vi "Loop_ACT_Drive.vi"() -> ()   [LabVIEW 2017]
uses:
  TypeDef/CLUSTER_Drive_HW_SRX_Status.ctl
  TypeDef/CLUSTER_4296_SRX_Status.ctl
  TypeDef/CLUSTER_SRX_Status Data.ctl
  TypeDef/CLUSTER_SRX_Encoder Data.ctl
  TypeDef/CLUSTER_SRX_PWM Data.ctl
  TypeDef/CLUSTER_SRX_Analog Data.ctl
  TypeDef/CLUSTER_SRX_Limit Switch Data.ctl
  TypeDef/CLUSTER_SRX_Profile Data.ctl
  TypeDef/ENUM_Drive_ACT Loop_Mode.ctl
  TypeDef/CLUSTER_Left and Right.ctl
  System Drivers/Phoenix-LabVIEW/Motor Controller/Controls/CTRE_Phoenix_MotorControl_FeedbackDevice.ctl
  System Drivers/Phoenix-LabVIEW/Motor Controller/Controls/CTRE_Phoenix_MotorControl_NeutralMode.ctl
  <vilib>/Rock Robotics/WPI/RobotDrive/WPI_RobotDriveOpen4MotorWithExistingMotors.vi
  _SHARE ALL/Global Share All/Global_STOP.vi
  Global_SM Write_Data Out.vi
  Global_ACT Write_Data Out.vi
  Drive Code/RoboRio Code/Systems/WCDrive2018/WCDrive2018.lvlib
  Drive Code/RoboRio Code/Systems/WCDrive2018/Cluster_WCDrive_SetupData.ctl
panel:
  in  "Zero Encoder":bool
  in  "D":dbl
  in  "I":dbl
  in  "P":dbl
  out "Right Data":dbl
  out "Left Data":dbl
  out "Cycle Time (S)":dbl format="%.3g"
  in  "Target Time(ms)":u32=50
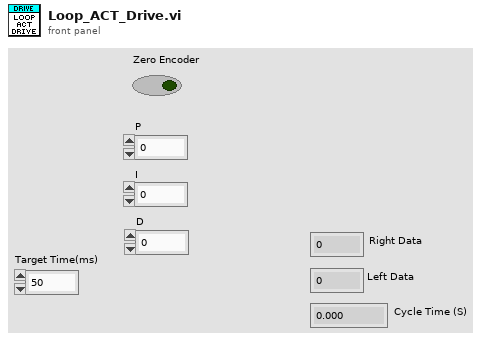
[diagram p1: front panel]
types:
  T1 = typedef "CTRE_Phoenix_MotorControl_NeutralMode.ctl" = enum8{"EEPROMSetting", "Override to Coast", "Override to Brake"}
  T2 = typedef "CTRE_Phoenix_MotorControl_FeedbackDevice.ctl" = i8
  T3 = typedef "CLUSTER_Left and Right.ctl" = cluster{"Left":dbl, "Right":dbl}
  T4 = typedef "ENUM_Drive_ACT Loop_Mode.ctl" = enum16{"Stop", "Position", "VBus", "Profile"}
  T5 = typedef "CLUSTER_Drive_HW_SRX_Status.ctl" = cluster{"Rear Left":T6, "Rear Right":T6, "Front Left":T6, "Front Right":T6}
  T6 = typedef "CLUSTER_4296_SRX_Status.ctl" = cluster{"Status":T7, "Encoder":T8, "PWM ":T9, "Analog":T10, "Limit Switches":T11, "Profile":T12}
  T7 = typedef "CLUSTER_SRX_Status Data.ctl" = cluster{"Module Enabled":bool, "Current Profile Slot Select":dbl, "Brake is Enabled":bool, "Applied Throttle":dbl, "Current":dbl, "Battery Voltage":dbl, "Sticky Fault - Under Voltage":bool, "Temperature (C)":dbl, "Sticky Fault - Over Temp":bool, "CAN Error":errorcluster, "Control 5 Is Supported":bool}
  T8 = typedef "CLUSTER_SRX_Encoder Data.ctl" = cluster{"Closed Loop Error":dbl, "Sensor Position":dbl, "Sensor Velocity":dbl, "Encoder Position":dbl, "Encoder Velocity":dbl, "Encoder Index Count":dbl, "Encoder A Pin State":bool, "Encoder B Pin State":bool, "Encoder Index Pin State":bool, "Pos Div 8":bool, "Vel Div 4":bool}
  T9 = typedef "CLUSTER_SRX_PWM Data.ctl" = cluster{"Closed Loop Error":dbl, "Pulse Width Position":i32, "Pulse Width Velocity":i32, "Pulse Width Rise To Rise (us)":i32, "Pulse Width Rise To Fall (us)":i32}
  T10 = typedef "CLUSTER_SRX_Analog Data.ctl" = cluster{"Closed Loop Error":dbl, "Analog In":dbl, "Analog In Velocity":dbl}
  T11 = typedef "CLUSTER_SRX_Limit Switch Data.ctl" = cluster{"Forward Limit Switch Closed":bool, "Reverse Limit Switch Closed":bool, "Sticky Fault - Forward Limit":bool, "Sticky Fault - Reverse Limit":bool, "Sticky Fault - Forward Soft Limit":bool, "Sticky Fault - Reverse Soft Limit":bool}
  T12 = typedef "CLUSTER_SRX_Profile Data.ctl" = cluster{"Mot Prof Active Is Under Run":bool, "Mot Prof Active Has Under Run":bool, "Mot Prof Active Is Last":bool, "Mot Prof Active Velocity Only":bool, "Mot Prof Active Is Valid":bool, "Mot Prof Buffer Is Full":bool, "Mot Prof Active Profile Slot Select":i32, "Mot Prof NextID":i32, "Mot Prof Count":i32, "Mot Prof Active Velocity":dbl, "Mot Prof Active Position":dbl, "Mot Prof Output Enable":i32}
  T13 = typedef "Cluster_WCDrive_SetupData.ctl" = cluster{"Left Master":u8, "Invert Left Master":bool, "Left Slave":u8, "Invert Left Slave":bool, "Right Master":u8, "Invert Right Master":bool, "Right Slave":u8, "Invert Right Slave":bool, "Invert Left Encoder":bool, "Invert Right Encoder":bool}
  T14 = typedef "WPI_MotorControlDeviceRef.ctl" = cluster{"DeviceStatus":errorcluster, "Type":T15, "PWM":cluster{"PWM Channel":T16, "DeadBand":T17}, "CAN":cluster{"Device Number":u8, "SetOutput VI Ref":variant, "GetOutput VI Ref":variant, "Enable VI Ref":variant, "Disable VI Ref":variant, "Data":variant}, "Invert":bool, "DIO PWM":cluster{"PWM \"Enable\" Channel":T16, "DIOChannel":T18, "PWM Rate":dbl}}
  T15 = typedef "WPI_MotorControlType.ctl" = enum16{"PWM", "CAN", "DIO PWM"}
  T16 = typedef "FPGA_DIOPWMChannel.ctl" = enum8{"PWM 0", "PWM 1", "PWM 2", "PWM 3", "PWM 4", "PWM 5", "PWM 6", "PWM 7", "PWM 8", "PWM 9", "PWM MXP 0", "PWM MXP 1", "PWM MXP 2", "PWM MXP 3", "PWM MXP 4", "PWM MXP 5", "PWM MXP 6", "PWM MXP 7", "PWM MXP 8", "PWM MXP 9", "Invalid"}
  T17 = typedef "WPI_PWMDeadband.ctl" = cluster{"Name":string, "maxPositivePwm":i32, "minPositivePwm":i32, "centerPwm":i32, "maxNegativePwm":i32, "minNegativePwm":i32, "angularRange":u16}
  T18 = typedef "FPGA_DIOChannel.ctl" = enum8{"DIO 0", "DIO 1", "DIO 2", "DIO 3", "DIO 4", "DIO 5", "DIO 6", "DIO 7", "DIO 8", "DIO 9", "DIO MXP 0", "DIO MXP 1", "DIO MXP 2", "DIO MXP 3", "DIO MXP 4", "DIO MXP 5", "DIO MXP 6", "DIO MXP 7", "DIO MXP 8", "DIO MXP 9", "DIO MXP 10", "DIO MXP 11", "DIO MXP 12", "DIO MXP 13", "DIO MXP 14", "DIO MXP 15", "SPI Port CS1", "SPI Port CS2", "SPI Port CS3", "SPI Port MISO", "SPI Port MOSI", "Invalid"}
  T19 = typedef "WPI_RobotDriveDevRef.ctl" = cluster{"DevStatus":errorcluster, "Motors[]":T14[], "Square Inputs":bool, "Max Output":dbl}
  T20 = cluster{"RobotDriveDevRef":T19, "Target Time(ms)":u32, "Current Time":timestamp, "Previous Time":timestamp, "Cycle Time (S)":dbl, "SRX_Status":T5, "Mode":T4, "VBus":T3, "Cruise RPM":dbl, "MAX Velocity\n":dbl, "Encoder Target Position":i32, "Zero Encoder":bool}
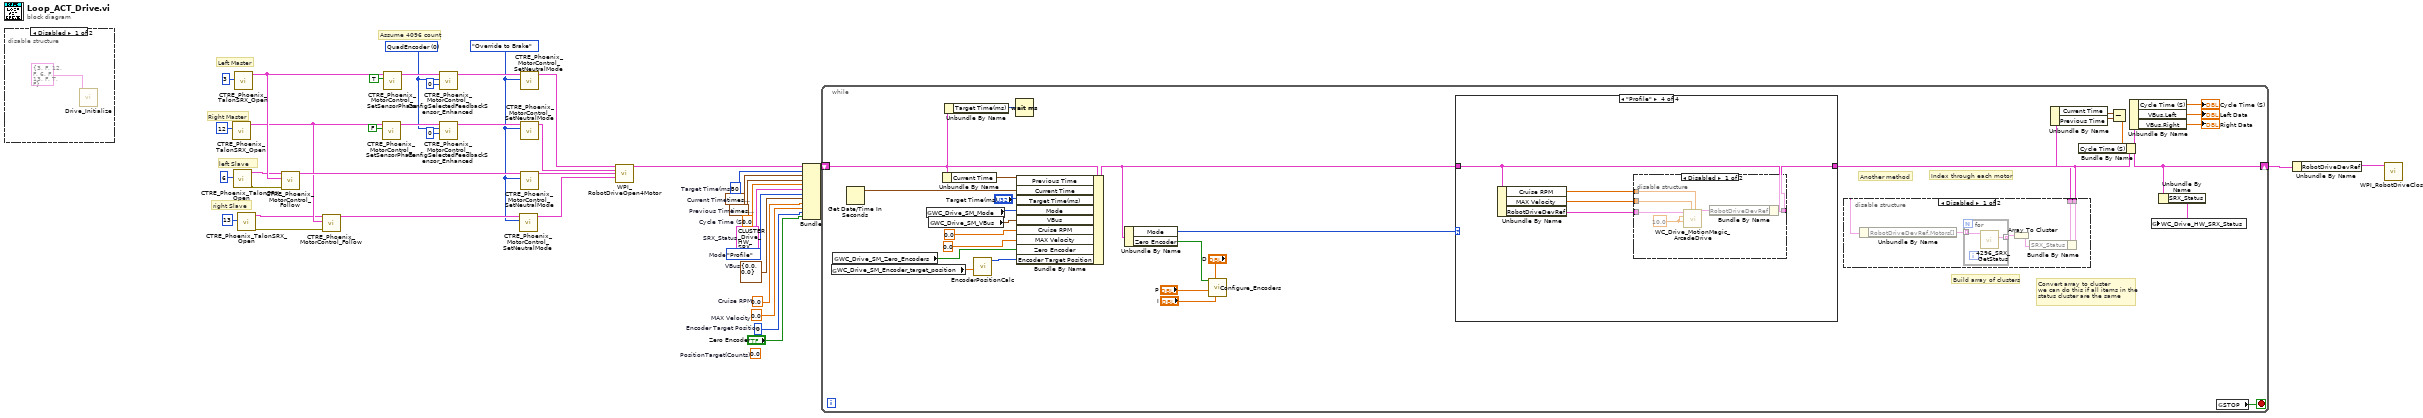
[diagram p0: block diagram]
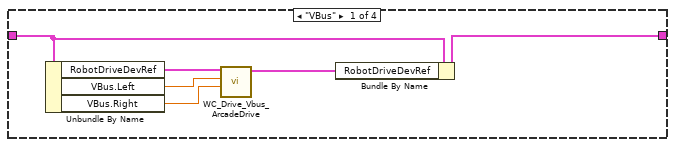
[diagram p4: hidden frame]
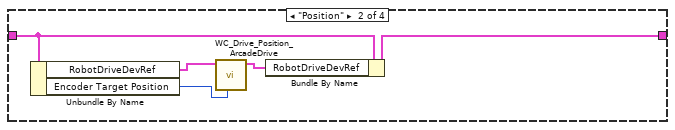
[diagram p5: hidden frame]
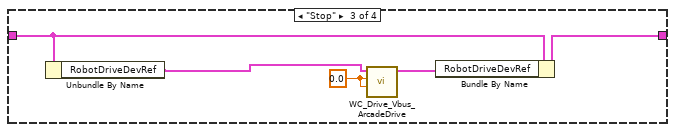
[diagram p6: hidden frame]
diagram:
  w14 = CTRE_Phoenix_MotorControl_NeutralMode."Override to Brake" ("Motor Control Neutral Mode")
  w17 = T2 0 items=["None"=-1, "QuadEncoder"=0, "Analog"=2, "Tachometer"=4, "Pulse Width Encoded Position"=8, "Sensor Sum (S0 + S1)"=9, "Sensor Difference (D0 - D1)"=10, "Remote Source 0"=11, "Remote Source 1"=12, "Software Emulated"=15] ("Feedback Device")
  (unwired) 0.0  # PositionTarget(Counts)
  w29 = 0  # Encoder Target Position
  w30 = 0.0  # MAX Velocity
  w31 = 0.0  # Cruise RPM
  w32 = T3 {"Left"=0.0, "Right"=0.0}  # VBus
  w33 = ENUM_Drive_ACT_Loop_Mode."Profile"  # Mode
  w34 = T5 {"Rear Left"={"Status"={"Module Enabled"=FALSE, "Current Profile Slot Select"=0.0, "Brake is Enabled"=FALSE, "Applied Throttle"=0.0, "Current"=0.0, "Battery Voltage"=0.0, "Sticky Fault - Under Voltage"=FALSE, "Temperature (C)"=0.0, "Sticky Fault - Over Temp"=FALSE, "CAN Error"={"status"=FALSE, "code"=0, "source"=""}, "Control 5 Is Supported"=FALSE}, "Encoder"={"Closed Loop Error"=0.0, "Sensor Position"=0.0, "Sensor Velocity"=0.0, "Encoder Position"=0.0, "Encoder Velocity"=0.0, "Encoder Index Count"=0.0, "Encoder A Pin State"=FALSE, "Encoder B Pin State"=FALSE, "Encoder Index Pin State"=FALSE, "Pos Div 8"=FALSE, "Vel Div 4"=FALSE}, "PWM "={"Closed Loop Error"=0.0, "Pulse Width Position"=0, "Pulse Width Velocity"=0, "Pulse Width Rise To Rise (us)"=0, "Pulse Width Rise To Fall (us)"=0}, "Analog"={"Closed Loop Error"=0.0, "Analog In"=0.0, "Analog In Velocity"=0.0}, "Limit Switches"={"Forward Limit Switch Closed"=FALSE, "Reverse Limit Switch Closed"=FALSE, "Sticky Fault - Forward Limit"=FALSE, "Sticky Fault - Reverse Limit"=FALSE, "Sticky Fault - Forward Soft Limit"=FALSE, "Sticky Fault - Reverse Soft Limit"=FALSE}, "Profile"={"Mot Prof Active Is Under Run"=FALSE, "Mot Prof Active Has Under Run"=FALSE, "Mot Prof Active Is Last"=FALSE, "Mot Prof Active Velocity Only"=FALSE, "Mot Prof Active Is Valid"=FALSE, "Mot Prof Buffer Is Full"=FALSE, "Mot Prof Active Profile Slot Select"=0, "Mot Prof NextID"=0, "Mot Prof Count"=0, "Mot Prof Active Velocity"=0.0, "Mot Prof Active Position"=0.0, "Mot Prof Output Enable"=0}}, "Rear Right"={"Status"={"Module Enabled"=FALSE, "Current Profile Slot Select"=0.0, "Brake is Enabled"=FALSE, "Applied Throttle"=0.0, "Current"=0.0, "Battery Voltage"=0.0, "Sticky Fault - Under Voltage"=FALSE, "Temperature (C)"=0.0, "Sticky Fault - Over Temp"=FALSE, "CAN Error"={"status"=FALSE, "code"=0, "source"=""}, "Control 5 Is Supported"=FALSE}, "Encoder"={"Closed Loop Error"=0.0, "Sensor Position"=0.0, "Sensor Velocity"=0.0, "Encoder Position"=0.0, "Encoder Velocity"=0.0, "Encoder Index Count"=0.0, "Encoder A Pin State"=FALSE, "Encoder B Pin State"=FALSE, "Encoder Index Pin State"=FALSE, "Pos Div 8"=FALSE, "Vel Div 4"=FALSE}, "PWM "={"Closed Loop Error"=0.0, "Pulse Width Position"=0, "Pulse Width Velocity"=0, "Pulse Width Rise To Rise (us)"=0, "Pulse Width Rise To Fall (us)"=0}, "Analog"={"Closed Loop Error"=0.0, "Analog In"=0.0, "Analog In Velocity"=0.0}, "Limit Switches"={"Forward Limit Switch Closed"=FALSE, "Reverse Limit Switch Closed"=FALSE, "Sticky Fault - Forward Limit"=FALSE, "Sticky Fault - Reverse Limit"=FALSE, "Sticky Fault - Forward Soft Limit"=FALSE, "Sticky Fault - Reverse Soft Limit"=FALSE}, "Profile"={"Mot Prof Active Is Under Run"=FALSE, "Mot Prof Active Has Under Run"=FALSE, "Mot Prof Active Is Last"=FALSE, "Mot Prof Active Velocity Only"=FALSE, "Mot Prof Active Is Valid"=FALSE, "Mot Prof Buffer Is Full"=FALSE, "Mot Prof Active Profile Slot Select"=0, "Mot Prof NextID"=0, "Mot Prof Count"=0, "Mot Prof Active Velocity"=0.0, "Mot Prof Active Position"=0.0, "Mot Prof Output Enable"=0}}, "Front Left"={"Status"={"Module Enabled"=FALSE, "Current Profile Slot Select"=0.0, "Brake is Enabled"=FALSE, "Applied Throttle"=0.0, "Current"=0.0, "Battery Voltage"=0.0, "Sticky Fault - Under Voltage"=FALSE, "Temperature (C)"=0.0, "Sticky Fault - Over Temp"=FALSE, "CAN Error"={"status"=FALSE, "code"=0, "source"=""}, "Control 5 Is Supported"=FALSE}, "Encoder"={"Closed Loop Error"=0.0, "Sensor Position"=0.0, "Sensor Velocity"=0.0, "Encoder Position"=0.0, "Encoder Velocity"=0.0, "Encoder Index Count"=0.0, "Encoder A Pin State"=FALSE, "Encoder B Pin State"=FALSE, "Encoder Index Pin State"=FALSE, "Pos Div 8"=FALSE, "Vel Div 4"=FALSE}, "PWM "={"Closed Loop Error"=0.0, "Pulse Width Position"=0, "Pulse Width Velocity"=0, "Pulse Width Rise To Rise (us)"=0, "Pulse Width Rise To Fall (us)"=0}, "Analog"={"Closed Loop Error"=0.0, "Analog In"=0.0, "Analog In Velocity"=0.0}, "Limit Switches"={"Forward Limit Switch Closed"=FALSE, "Reverse Limit Switch Closed"=FALSE, "Sticky Fault - Forward Limit"=FALSE, "Sticky Fault - Reverse Limit"=FALSE, "Sticky Fault - Forward Soft Limit"=FALSE, "Sticky Fault - Reverse Soft Limit"=FALSE}, "Profile"={"Mot Prof Active Is Under Run"=FALSE, "Mot Prof Active Has Under Run"=FALSE, "Mot Prof Active Is Last"=FALSE, "Mot Prof Active Velocity Only"=FALSE, "Mot Prof Active Is Valid"=FALSE, "Mot Prof Buffer Is Full"=FALSE, "Mot Prof Active Profile Slot Select"=0, "Mot Prof NextID"=0, "Mot Prof Count"=0, "Mot Prof Active Velocity"=0.0, "Mot Prof Active Position"=0.0, "Mot Prof Output Enable"=0}}, "Front Right"={"Status"={"Module Enabled"=FALSE, "Current Profile Slot Select"=0.0, "Brake is Enabled"=FALSE, "Applied Throttle"=0.0, "Current"=0.0, "Battery Voltage"=0.0, "Sticky Fault - Under Voltage"=FALSE, "Temperature (C)"=0.0, "Sticky Fault - Over Temp"=FALSE, "CAN Error"={"status"=FALSE, "code"=0, "source"=""}, "Control 5 Is Supported"=FALSE}, "Encoder"={"Closed Loop Error"=0.0, "Sensor Position"=0.0, "Sensor Velocity"=0.0, "Encoder Position"=0.0, "Encoder Velocity"=0.0, "Encoder Index Count"=0.0, "Encoder A Pin State"=FALSE, "Encoder B Pin State"=FALSE, "Encoder Index Pin State"=FALSE, "Pos Div 8"=FALSE, "Vel Div 4"=FALSE}, "PWM "={"Closed Loop Error"=0.0, "Pulse Width Position"=0, "Pulse Width Velocity"=0, "Pulse Width Rise To Rise (us)"=0, "Pulse Width Rise To Fall (us)"=0}, "Analog"={"Closed Loop Error"=0.0, "Analog In"=0.0, "Analog In Velocity"=0.0}, "Limit Switches"={"Forward Limit Switch Closed"=FALSE, "Reverse Limit Switch Closed"=FALSE, "Sticky Fault - Forward Limit"=FALSE, "Sticky Fault - Reverse Limit"=FALSE, "Sticky Fault - Forward Soft Limit"=FALSE, "Sticky Fault - Reverse Soft Limit"=FALSE}, "Profile"={"Mot Prof Active Is Under Run"=FALSE, "Mot Prof Active Has Under Run"=FALSE, "Mot Prof Active Is Last"=FALSE, "Mot Prof Active Velocity Only"=FALSE, "Mot Prof Active Is Valid"=FALSE, "Mot Prof Buffer Is Full"=FALSE, "Mot Prof Active Profile Slot Select"=0, "Mot Prof NextID"=0, "Mot Prof Count"=0, "Mot Prof Active Velocity"=0.0, "Mot Prof Active Position"=0.0, "Mot Prof Output Enable"=0}}}  # SRX_Status
  w36 = 0.0  # Cycle Time (S)
  w41 = timestamp(0 s since 1904-01-01)  # Previous Time
  w40 = timestamp(0 s since 1904-01-01)  # Current Time
  w39 = u32 50  # Target Time(ms)
  # "right Slave"
  # "Assume 4096 count"
  # "left Slave"
  # "Right Master"
  # "Left Master"
  n1 = disable-structure shown="Disabled" {
    frame Disabled {
      n2 = call "Drive_Initialize.vi"("HW SETUP_WC Drive"=T13 {"Left Master"=3, "Invert Left Master"=FALSE, "Left Slave"=12, "Invert Left Slave"=FALSE, "Right Master"=6, "Invert Right Master"=FALSE, "Right Slave"=13, "Invert Right Slave"=FALSE, "Invert Left Encoder"=TRUE, "Invert Right Encoder"=FALSE}) -> ()  [unwired: 10 in, 1 out]
    }
    frame Enabled {
    }
  }
  n3 = call "CTRE_Phoenix_TalonSRX_Open.vi"("Device Number"=u8 12) -> ("CAN Talon SRX Ref"=w21:T14)  [unwired: 9 in, 1 out]
  n4 = call "CTRE_Phoenix_TalonSRX_Open.vi"("Device Number"=u8 6) -> ("error out"=w10:errorcluster, "CAN Talon SRX Ref"=w11:T14)  [unwired: 9 in]
  n5 = call "CTRE_Phoenix_TalonSRX_Open.vi"("Device Number"=u8 3) -> ("CAN Talon SRX Ref"=w23:T14)  [unwired: 9 in, 1 out]
  n6 = call "CTRE_Phoenix_TalonSRX_Open.vi"("Device Number"=u8 13) -> ("error out"=w8:errorcluster, "CAN Talon SRX Ref"=w9:T14)  [unwired: 9 in]
  n7 = call "CTRE_Phoenix_MotorControl_Follow.vi"("error in (no error)"=w10, "Master Controller to Follow"=w23, "PhoenixMotorControlDevRef"=w11) -> ("PhoenixMotorControlDevRef"=w22:T14)  [unwired: 7 in, 1 out]
  n8 = call "CTRE_Phoenix_MotorControl_Follow.vi"("error in (no error)"=w8, "Master Controller to Follow"=w21, "PhoenixMotorControlDevRef"=w9) -> ("PhoenixMotorControlDevRef"=w20:T14)  [unwired: 7 in, 1 out]
  n9 = call "CTRE_Phoenix_MotorControl_SetSensorPhase.vi"("PhaseSensor"=FALSE, "PhoenixMotorControlDevRef"=w21) -> ("PhoenixMotorControlDevRef"=w18:T14)  [unwired: 8 in, 1 out]
  n10 = call "CTRE_Phoenix_MotorControl_SetSensorPhase.vi"("PhaseSensor"=TRUE, "PhoenixMotorControlDevRef"=w23) -> ("PhoenixMotorControlDevRef"=w19:T14)  [unwired: 8 in, 1 out]
  n11 = call "CTRE_Phoenix_MotorControl_ConfigSelectedFeedbackSensor_Enhanced.vi"("pidLoopIdx"=0, "Feedback Device"=w17, "PhoenixMotorControlDevRef"=w19) -> ("PhoenixMotorControlDevRef"=w16:T14)  [unwired: 7 in, 1 out]
  n12 = call "CTRE_Phoenix_MotorControl_ConfigSelectedFeedbackSensor_Enhanced.vi"("pidLoopIdx"=0, "Feedback Device"=w17, "PhoenixMotorControlDevRef"=w18) -> ("PhoenixMotorControlDevRef"=w15:T14)  [unwired: 7 in, 1 out]
  n13 = call "CTRE_Phoenix_MotorControl_SetNeutralMode.vi"("Motor Control Neutral Mode"=w14, "PhoenixMotorControlDevRef"=w20) -> ("PhoenixMotorControlDevRef"=w27:T14)  [unwired: 8 in, 1 out]
  n14 = call "CTRE_Phoenix_MotorControl_SetNeutralMode.vi"("Motor Control Neutral Mode"=w14, "PhoenixMotorControlDevRef"=w22) -> ("PhoenixMotorControlDevRef"=w26:T14)  [unwired: 8 in, 1 out]
  n15 = call "CTRE_Phoenix_MotorControl_SetNeutralMode.vi"("Motor Control Neutral Mode"=w14, "PhoenixMotorControlDevRef"=w16) -> ("PhoenixMotorControlDevRef"=w24:T14)  [unwired: 8 in, 1 out]
  n16 = call "CTRE_Phoenix_MotorControl_SetNeutralMode.vi"("Motor Control Neutral Mode"=w14, "PhoenixMotorControlDevRef"=w15) -> ("PhoenixMotorControlDevRef"=w25:T14)  [unwired: 8 in, 1 out]
  n17 = call-poly <vilib>:"WPI_RobotDriveOpen4Motor.vi"("Rear Left Motor Dev Ref"=w24, "Rear Right Motor Dev Ref"=w25, "Front Left Motor Dev Ref"=w26, "Front Right Motor Dev Ref"=w27) -> ("RobotDriveDevRef"=w3:T19)  [unwired: 10 in, 1 out]
  n18 = Bundle("RobotDriveDevRef"=w3, "Target Time(ms)"=w39, "Current Time"=w40, "Previous Time"=w41, "Cycle Time (S)"=w36, "SRX_Status"=w34, "Mode"=w33, "VBus"=w32, "Cruise RPM"=w31, "MAX Velocity"=w30, "Encoder Target Position"=w29, "Zero Encoder"="Zero Encoder") -> (w38:T20)  [unwired: 1 in]
  n19 = while {
    shift-right: [w57] -> w37
    shift-left: w38 -> [w44]
    stop <- w71 stop-if-true
    # "Build array of clusters"
    # "Convert array to cluster\nwe can do this if all items in the\nstatus cluster are the same"
    # "Index through each motor"
    # "Another method"
    n20 = global read "Global_SM Write_Data Out.vi" "WC_Drive_SM_Encoder_target_position"() -> (w45:dbl)
    n21 = global read "Global_SM Write_Data Out.vi" "WC_Drive_SM_Zero_Encoders"() -> (w47:bool)
    n22 = Get Date/Time In Seconds() -> (seconds since 1Jan1904=w70:timestamp)
    n23 = global read "Global_SM Write_Data Out.vi" "WC_Drive_SM_Mode"() -> (w60:T4)
    n24 = global read "Global_SM Write_Data Out.vi" "WC_Drive_SM_VBus"() -> (w54:T3)
    n25 = Unbundle By Name(w44) -> ("Current Time"=w69:timestamp)
    n26 = Unbundle By Name(w44) -> ("Target Time(ms)"=w65:u32)
    n27 = call "EncoderPositionCalc.vi"("PositionTarget(in)"=w45) -> ("PostionTarget(Counts)"=w46:i32)  [unwired: 10 in]
    n28 = Wait (ms)(milliseconds to wait=w65) -> ()  [unwired: 1 out]
    n29 = Bundle By Name(cluster=w44, "Previous Time"=w69, "Current Time"=w70, "Target Time(ms)"="Target Time(ms)", "Mode"=w60, "VBus"=w54, "Cruise RPM"=0.0, "MAX Velocity"=0.0, "Zero Encoder"=w47, "Encoder Target Position"=w46) -> (w43:T20)
    n30 = Unbundle By Name(w43) -> ("Mode"=w59:T4, "Zero Encoder"=w48:bool)
    n31 = call "Configure_Encoders.vi"("I"="I", "D"="D", "P"="P", "Zero Encoder"=w48) -> ()  [unwired: 8 in]
    n32 = case shown="\"Profile\"" w59 {
      tunnel: w43 -> [w82 w89 w94 w97]
      tunnel: [w81 w88 w93 w98] -> w55
      frame "VBus" {
        n33 = Unbundle By Name(w82) -> ("RobotDriveDevRef"=w80:T19, "VBus.Left"=w84:dbl, "VBus.Right"=w83:dbl)
        n34 = call "WC_Drive_Vbus_ArcadeDrive.vi"("Right Value"=w83, "Left Value"=w84, "RobotDriveDevRef"=w80) -> ("RobotDriveDevRef Out"=w79:T19)  [unwired: 7 in, 1 out]
        n35 = Bundle By Name(cluster=w82, "RobotDriveDevRef"=w79) -> (w81:T20)
      }
      frame "Position" {
        n36 = Unbundle By Name(w89) -> ("RobotDriveDevRef"=w86:T19, "Encoder Target Position"=w87:i32)
        n37 = call "WC_Drive_Position_ArcadeDrive.vi"("Encoder Target Position"=w87, "RobotDriveDevRef"=w86) -> ("RobotDriveDevRef Out"=w85:T19)  [unwired: 8 in, 1 out]
        n38 = Bundle By Name(cluster=w89, "RobotDriveDevRef"=w85) -> (w88:T20)
      }
      frame "Stop" {
        w91 = 0.0 ("X axis value")
        n39 = Unbundle By Name(w94) -> ("RobotDriveDevRef"=w92:T19)
        n40 = call "WC_Drive_Vbus_ArcadeDrive.vi"("Right Value"=w91, "Left Value"=w91, "RobotDriveDevRef"=w92) -> ("RobotDriveDevRef Out"=w90:T19)  [unwired: 7 in, 1 out]
        n41 = Bundle By Name(cluster=w94, "RobotDriveDevRef"=w90) -> (w93:T20)
      }
      frame "Profile" {
        n42 = Unbundle By Name(w97) -> ("Cruise RPM"=w96:dbl, "MAX Velocity"=w95:dbl, "RobotDriveDevRef"=w99:T19)
        n43 = disable-structure shown="Disabled" {
          disable-tunnel: w99 -> [w106 _]
          disable-tunnel: [w103 _] -> w98
          disable-tunnel: w97 -> [w102 _]
          disable-tunnel: w96 -> [w101 _]
          disable-tunnel: w95 -> [w100 _]
          frame Disabled {
            w105 = 10.0 ("X axis value")
            n44 = call "WC_Drive_MotionMagic_ArcadeDrive.vi"("Cruise RPM"=w101, "Max Velocity"=w100, "Right Value"=w105, "Left Value"=w105, "RobotDriveDevRef"=w106) -> ("RobotDriveDevRef Out"=w104:T19)  [unwired: 5 in, 1 out]
            n45 = Bundle By Name(cluster=w102, "RobotDriveDevRef"=w104) -> (w103:T20)
          }
          frame Enabled {
          }
        }
      }
    }
    n46 = disable-structure shown="Disabled" {
      disable-tunnel: [w76 _] -> w56
      disable-tunnel: w55 -> [w75 _]
      frame Disabled {
        n47 = Unbundle By Name(w75) -> ("RobotDriveDevRef.Motors[]"=w74:T14[])
        n48 = for {
          tunnel: w74 -> [w78] mode=indexing
          tunnel: [w77] -> w73 mode=indexing
          n49 = call "4296_SRX_GetStatus.vi"("CAN Talon SRX Ref"=w78) -> ("4296 SRX Status Out"=w77:T6)  [unwired: 8 in, 2 out]
        }
        n50 = Array To Cluster(array=w73) -> (cluster=w72:cluster{"[0]":T6, "[1]":T6, "[2]":T6, "[3]":T6})
        n51 = Bundle By Name(cluster=w75, "SRX_Status"=w72) -> (w76:T20)
      }
      frame Enabled {
      }
    }
    n52 = Unbundle By Name(w56) -> ("Current Time"=w68:timestamp, "Previous Time"=w67:timestamp)
    n53 = Subtract(x=w68, y=w67) -> (x-y=w58:dbl)
    n54 = Bundle By Name(cluster=w56, "Cycle Time (S)"=w58) -> (w57:T20)
    n55 = Unbundle By Name(w57) -> ("Cycle Time (S)"=→"Cycle Time (S)":dbl, "VBus.Left"=→"Left Data":dbl, "VBus.Right"=→"Right Data":dbl)
    n56 = Unbundle By Name(w57) -> ("SRX_Status"=w61:T5)
    n57 = global write "Global_ACT Write_Data Out.vi" "WC_Drive_HW_SRX_Status"(w61) -> ()
    n58 = global read "Global_STOP.vi" "STOP"() -> (w71:bool)
  }
  n59 = Unbundle By Name(w37) -> ("RobotDriveDevRef"=w35:T19)
  n60 = call <vilib>:"WPI_RobotDriveClose.vi"("RobotDriveDevRef"=w35) -> ()  [unwired: 10 in, 1 out]
